vi "calc_outer.vi"(11 "Qube":refnum<class "System.lvclass">) -> (3 "Qube":refnum<class "System.lvclass">)   [LabVIEW 2021, in "System.lvclass"]
uses:
  System.lvclass
  System.lvclass/System.ctl
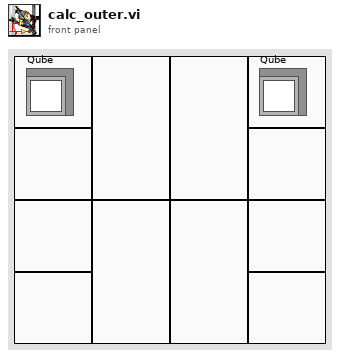
[diagram p1: front panel]
types:
  T1 = typedef "System.lvclass/mode.ctl" = enum16{"Control", "Identify"}
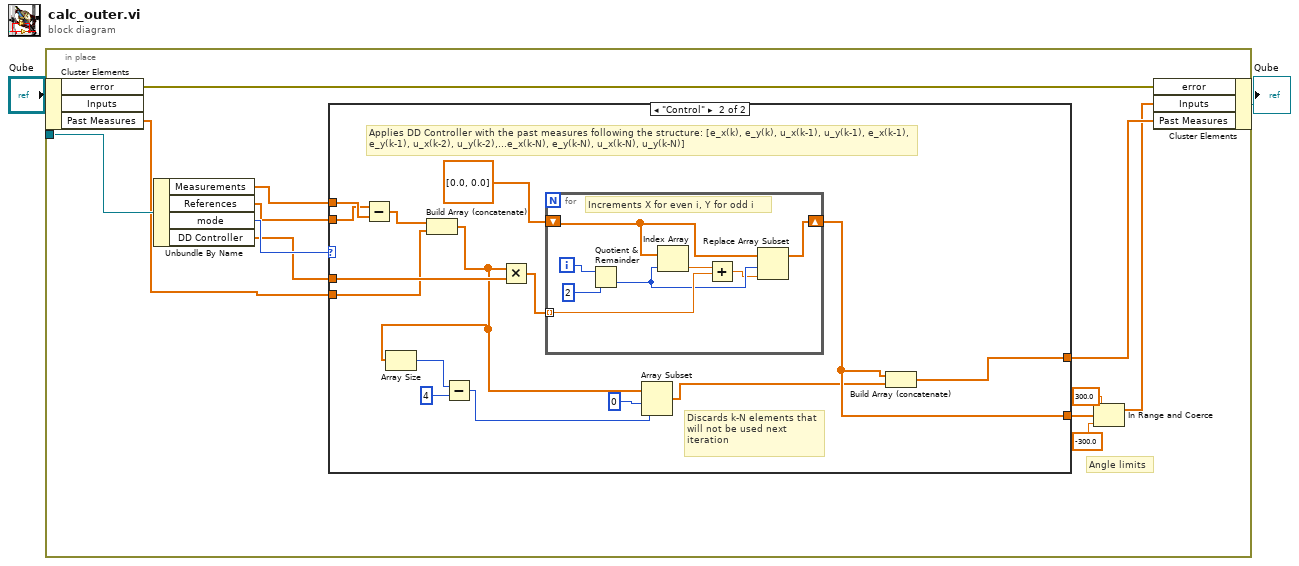
[diagram p0: block diagram]
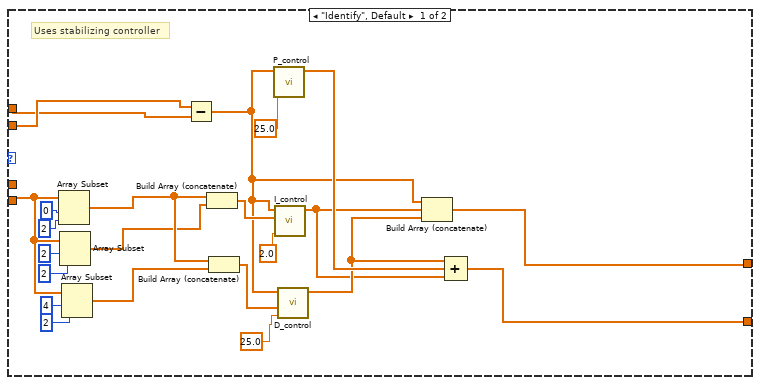
[diagram p2: hidden frame]
diagram:
  n1 = in-place {
    in-place-border: "Qube" -> [w12]
    # "Angle limits"
    n2 = in-place-cluster #1("Qube") -> ("error"=w14:errorcluster, "Past Measures"=w8:dbl[])  [unwired: 1 out]
    n3 = Unbundle By Name(w12) -> ("Measurements"=w10:dbl[], "References"=w11:dbl[], "mode"=w13:T1, "DD Controller"=w7:dbl[])
    n4 = case shown="\"Control\"" w13 {
      tunnel: w11 -> [w35 w51]
      tunnel: w10 -> [w31 w52]
      tunnel: [w32 w46] -> w5
      tunnel: [w33 w44] -> w9
      tunnel: w8 -> [w21 w42]
      tunnel: w7 -> [_ w49]
      frame "Identify", Default {
        # "Uses stabilizing controller"
        n5 = Array Subset(array=w21, index=0, length=2) -> (w30:dbl[])
        n6 = Array Subset(array=w21, index=2, length=2) -> (w29:dbl[])
        n7 = Array Subset(array=w21, index=4, length=2) -> (w28:dbl[])
        n8 = Subtract(x=w35, y=w31) -> (x-y=w19:dbl[])
        n9 = Build Array (concatenate)(w30, w29) -> (w20:dbl[])
        n10 = Build Array (concatenate)(w30, w28) -> (w18:dbl[])
        n11 = call "P_control.vi"("Kp"=25.0, "Feedback error"=w19) -> ("P control"=w36:dbl[])  [unwired: 9 in]
        n12 = call "I_control.vi"("Ki"=2.0, "Past measures"=w20, "Feedback error"=w19) -> ("I control"=w15:dbl[])  [unwired: 8 in]
        n13 = call "D_control.vi"("Kd"=25.0, "Past Measures"=w18, "Feedback error"=w19) -> ("D control"=w17:dbl[])  [unwired: 8 in]
        n14 = Build Array (concatenate)(w19, w15, w17) -> (w33:dbl[])
        n15 = Compound Arithmetic op=ADD(w17, w36, w15) -> (w32:dbl[])
      }
      frame "Control" {
        # "Discards k-N elements that will not be used next iteration"
        # "Applies DD Controller with the past measures following the structure: [e_x(k), e_y(k), u_x(k-1), u_y(k-1), e_x(k-1), e_y(k-1), u_x(k-2), u_y(k-2),...e_x(k-N), e_y(k-N), u_x(k-N), u_y(k-N)]"
        n16 = Subtract(x=w51, y=w52) -> (x-y=w50:dbl[])
        n17 = Build Array (concatenate)(w50, w42) -> (w38:dbl[])
        n18 = Array Size(array=w38) -> (size(s)=w41:i32)
        n19 = Subtract(x=w41, y=4) -> (x-y=w39:i32)
        n20 = Multiply(x=w38, y=w49) -> (x*y=w47:dbl[])
        n21 = for {
          shift-right: [w53] -> w46
          shift-left: dbl[] [0.0, 0.0] -> [w56]
          tunnel: w47 -> [w57] mode=indexing
          i -> [w60]
          # "Increments X for even i, Y for odd i"
          n22 = Quotient & Remainder(x=w60, y=2) -> (floor(x/y)=w55:i32)  [unwired: 1 out]
          n23 = Index Array(array=w56, index=w55) -> (element=w58:dbl)
          n24 = Add(x=w58, y=w57) -> (x+y=w54:dbl)
          n25 = Replace Array Subset(array=w56, new element=w54, index=w55) -> (w53:dbl[])
        }
        n26 = Array Subset(array=w38, index=0, length=w39) -> (w45:dbl[])
        n27 = Build Array (concatenate)(w46, w45) -> (w44:dbl[])
      }
    }
    n28 = In Range and Coerce(upper limit=300.0, x=w5, lower limit=-300.0) -> (coerced(x)=w6:dbl[])  [unwired: 1 out]
    n29 = in-place-cluster #1("error"=w14, "Inputs"=w6, "Past Measures"=w9) -> (→"Qube":refnum<class "System.lvclass">)
  }
